vi "WRP Get Error String.vi"(11 "index":i32) -> (1 "Return code":i32, 2 "size out":i32, 3 "value":string)   [LabVIEW 2018, in "SesWrapper.lvlib"]
uses:
  SesWrapper/SesWrapper.lvlib
  build/Debug/SESWrapper.dll
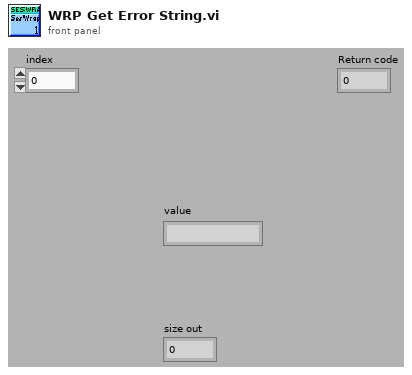
[diagram p1: front panel]
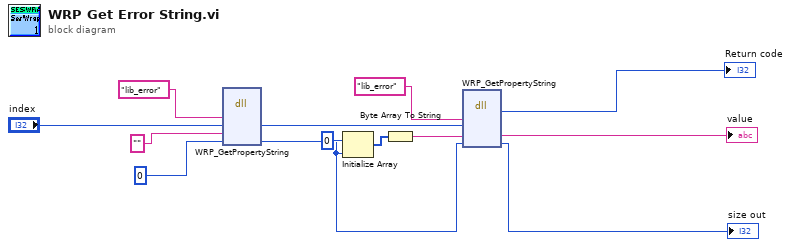
[diagram p0: block diagram]
diagram:
  n1 = dll-call lib="C:/Development/svn/seswrapper-lib/build/Debug/SESWrapper.*" fn="WRP_GetPropertyString"("property"="lib_error", "index"="index", "value"="", "size"=0) -> ("index"=w3:i32, "size"=w6:i32)  [unwired: 6 in, 2 out]
  n2 = Initialize Array(u8 0 ("element"), w6) -> (w13:u8[])
  n3 = Byte Array To String(unsigned byte array=w13) -> (string=w12:string)
  n4 = dll-call lib="C:/Development/svn/seswrapper-lib/build/Debug/SESWrapper.*" fn="WRP_GetPropertyString"("property"="lib_error", "index"=w3, "value"=w12, "size"=w6) -> (→"Return code":i32, "value"=→"value":string, "size"=→"size out":i32)  [unwired: 5 in, 2 out]
